vi "Add Mode Code.vi"(4 "create timestamp channel":bool, 6 "parameters":T2(array[cluster]), 7 "mode code":u16=1, 8 "error in":errorcluster, 9 "terminals":cluster{"Rx":T3, "Tx":T3}, 10 "name":string, 11 "port in":T5 format="%.0x") -> (0 "error out":errorcluster, 3 "port out":T5 format="%.0x")   [LabVIEW 2020, in "AIM MIL-STD-1553 Scripting.lvlib"]
uses:
  AIM MIL-STD-1553 Scripting.lvlib
  Shared/Address.ctl
  Shared/Terminal Endpoint.ctl
  Shared/Message Type.ctl
  Constants.vi
  <vilib>/NI VeriStand/Custom Device API/Custom Device Item Ref.ctl
  <vilib>/NI VeriStand/Custom Device API/Custom Device API.lvlib
  Shared/Parameter Definition.ctl
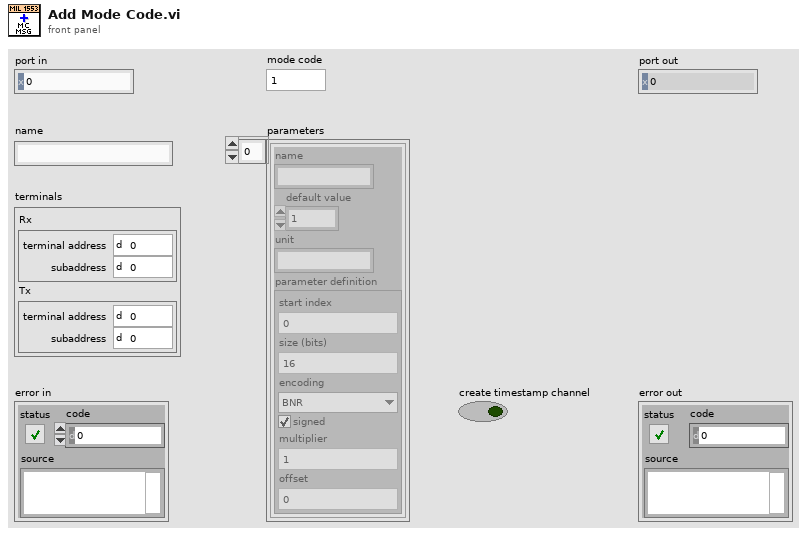
[diagram p1: front panel]
types:
  T1 = typedef "Parameter Definition.ctl" = cluster{"start index":i32, "size (bits)":i32, "encoding":enum16{"BNR", "BCD", "Discrete"}, "signed":bool, "multiplier":dbl, "offset":dbl}
  T2 = cluster{"name":string, "default value":dbl, "unit":string, "parameter definition":T1}[]
  T3 = typedef "Terminal Endpoint.ctl" = cluster{"terminal address":T4, "subaddress":T4}
  T4 = typedef "Address.ctl" = u16
  T5 = typedef "Custom Device API.lvlib/Custom Device Item Ref.ctl" = u64
  T6 = typedef "Message Type.ctl" = string
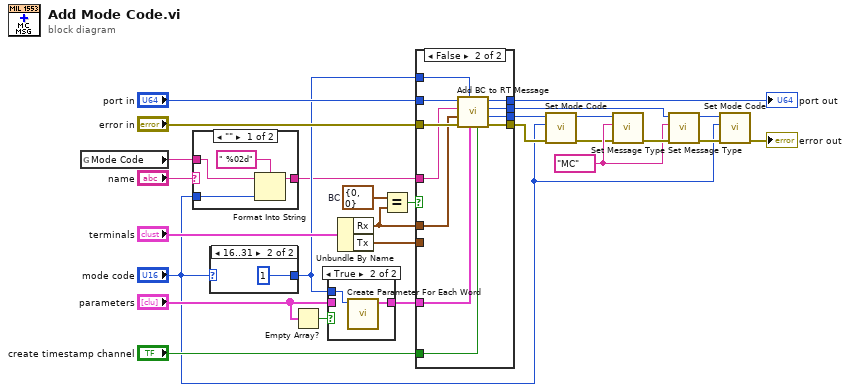
[diagram p0: block diagram]
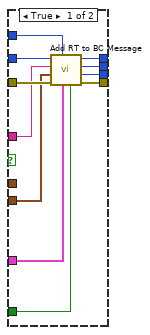
[diagram p3: hidden frame]
diagram:
  w10 = T6 "MC" ("message type")
  w24 = T3 {"terminal address"=0, "subaddress"=0}  # BC
  n1 = global read "Constants.vi" "Mode Code"() -> (w1:string)
  n2 = case shown="\"\"" "name" {
    selector: "name" -> [_ w32]
    tunnel: [w31 w32] -> w13
    tunnel: "mode code" -> [w30 _]
    tunnel: w1 -> [w28 _]
    frame "" {
      n3 = Format Into String(format string=" %02d", initial string=w28, w30) -> (resulting string=w31:string)  [unwired: 1 in, 1 out]
    }
    frame Default {
    }
  }
  n4 = case shown="16..31" "mode code" {
    tunnel: [_ u16 1 ("mode code")] -> w16
    frame Default {
    }
    frame 16..31 {
    }
  }
  n5 = Empty Array?(array="parameters") -> (empty?=w27:bool)
  n6 = case shown="True" w27 {
    tunnel: w16 -> [_ w36]
    tunnel: "parameters" -> [w34 _]
    tunnel: [w34 w35] -> w19
    frame False {
    }
    frame True {
      n7 = call "Create Parameter For Each Word.vi"("number of words"=w36) -> ("parameters"=w35:T2)  [unwired: 9 in, 1 out]
    }
  }
  n8 = Unbundle By Name("terminals") -> ("Rx"=w15:T3, "Tx"=w17:T3)
  n9 = Equal?(x=w24, y=w15) -> (x = y?=w23:bool)
  n10 = case shown="False" w23 {
    tunnel: "port in" -> [w47 w58]
    tunnel: "error in" -> [w46 w57]
    tunnel: [w45 w56] -> w9
    tunnel: [w44 w55] -> w20
    tunnel: w19 -> [w43 w54]
    tunnel: "create timestamp channel" -> [w42 w53]
    tunnel: w13 -> [w41 w52]
    tunnel: w17 -> [w40 _]
    tunnel: w16 -> [w39 w51]
    tunnel: w15 -> [_ w50]
    tunnel: [w38 w49] -> w11
    tunnel: [w37 w48] -> w8
    frame True {
      n11 = call "Add RT to BC Message.vi"("create timestamp channel"=w42, "parameters"=w43, "number of words"=w39, "error in"=w46, "Tx remote terminal"=w40, "name"=w41, "port in"=w47) -> ("error out"=w45:errorcluster, "BC message"=w37:T5, "RT message"=w38:T5, "port out"=w44:T5)  [unwired: 1 in]
    }
    frame False {
      n12 = call "Add BC to RT Message.vi"("create timestamp channel"=w53, "parameters"=w54, "number of words"=w51, "error in"=w57, "Rx remote terminal"=w50, "name"=w52, "port in"=w58) -> ("error out"=w56:errorcluster, "BC message"=w48:T5, "RT message"=w49:T5, "port out"=w55:T5)  [unwired: 1 in]
    }
  }
  "port out" <- w20
  n13 = call "Set Mode Code.vi"("error in"=w9, "mode code"="mode code", "message in"=w8) -> ("error out"=w7:errorcluster, "message out"=w6:T5)  [unwired: 7 in]
  n14 = call "Set Message Type.vi"("error in"=w7, "message type"=w10, "message in"=w6) -> ("error out"=w12:errorcluster)  [unwired: 7 in, 1 out]
  n15 = call "Set Message Type.vi"("error in"=w12, "message type"=w10, "message in"=w11) -> ("error out"=w4:errorcluster, "message out"=w5:T5)  [unwired: 7 in]
  n16 = call "Set Mode Code.vi"("error in"=w4, "mode code"="mode code", "message in"=w5) -> ("error out"=→"error out":errorcluster)  [unwired: 7 in, 1 out]
